vi "copy_method.vi"(6 "error in":errorcluster, 8 "name or relative path":string="config_data_cluster.ctl", 9 "new class reference in":refnum<vi>) -> (0 "error out":errorcluster, 3 "new class refernce out":refnum<vi>)   [LabVIEW 2010]
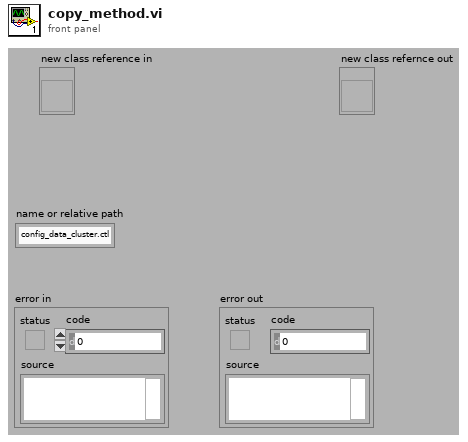
[diagram p1: front panel]
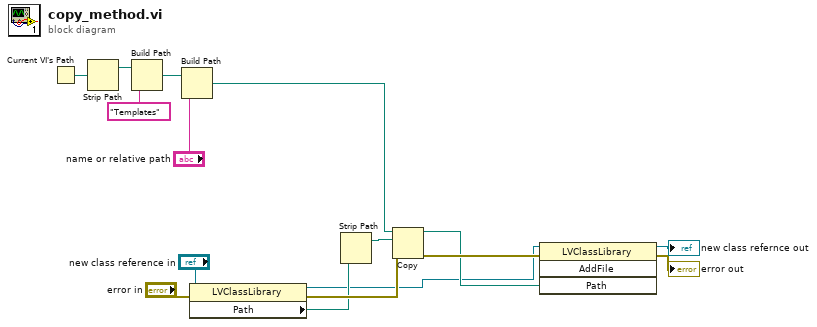
[diagram p0: block diagram]
diagram:
  n1 = Current VI's Path() -> (path=w12:path)
  n2 = Strip Path(path=w12) -> (stripped path=w11:path)  [unwired: 1 out]
  n3 = Build Path(base path=w11, name or relative path="Templates") -> (appended path=w9:path)
  n4 = Build Path(base path=w9, name or relative path="name or relative path") -> (appended path=w13:path)
  n5 = property class="LVClassLibrary"(reference="new class reference in", error in="error in") -> (reference out=w1:refnum<vi>, error out=w4:errorcluster, "Path"=w3:path)
  n6 = Strip Path(path=w3) -> (stripped path=w6:path)  [unwired: 1 out]
  n7 = Copy(8:w4, 10:w6, 11:w13) -> (0:w15:errorcluster, 3:w14:path)  [unwired: 2 in, 1 out]
  n8 = invoke on="Invoke Node" class="LVClassLibrary" method="AddFile"(reference=w1, error in=w15, "Path"=w14) -> (reference out=→"new class refernce out":refnum<vi>, error out=→"error out":errorcluster)  [unwired: 1 in, 2 out]
